vi "Input Items Write.vi"(4 "error in (no error)":errorcluster, 5 "Value":string[](array[string]), 6 "Container State":T4, 7 "Display State In":T1) -> (0 "error out":errorcluster, 3 "Display State Out":T1)   [LabVIEW 2020, in "PXISlotGP.xctl"]
uses:
  PXISlotGP.xctl
  <vilib>/_xctls/Container State.ctl
  State.ctl
  PXISlot XControl/Connector Type.ctl
  AOAIRefs.ctl
  <vilib>/_xctls/XControlSupport.lvlib
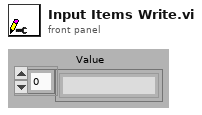
[diagram p1: front panel]
types:
  T1 = typedef "PXISlotGP.xctl/State.ctl" = cluster{"Connector Type":T2, "Hide unused":bool, "Trigger Visible":bool, "TabRef":refnum<vi>, "ConnRefs":refnum<vi>[], "PaneRef":refnum<vi>, "AOAIRefs":T3[], "TriggerRefs":refnum<vi>[], "check data":bool, "Name":string, "Events":cluster{"Type changed":refnum<user-event>}}
  T2 = typedef "Connector Type.ctl" = enum16{"None", "PXI-4461", "BNC-2110", "BNC-2090", "PXIe-4463", "PXIe-4464"}
  T3 = typedef "AOAIRefs.ctl" = cluster{"AORefs":refnum<vi>[], "AIRefs":refnum<vi>[]}
  T4 = typedef "XControlSupport.lvlib/Container State.ctl" = cluster{"Indicator?":bool, "Run Mode?":bool, " Refnum":refnum<vi>}
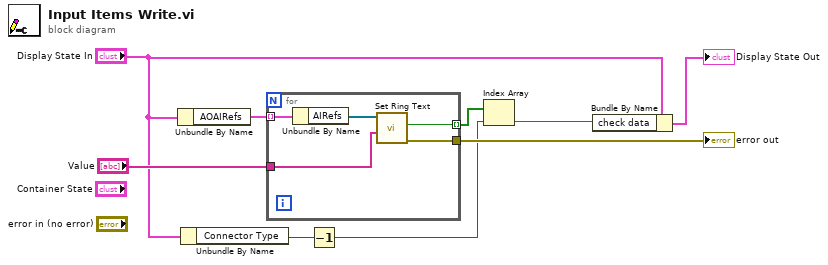
[diagram p0: block diagram]
diagram:
  n1 = Unbundle By Name("Display State In") -> ("AOAIRefs"=w9:T3[])
  n2 = Unbundle By Name("Display State In") -> ("Connector Type"=w3:T2)
  n3 = for {
    tunnel: w9 -> [w14] mode=indexing
    tunnel: "Value" -> [w12]
    tunnel: [w11] -> w7
    tunnel: [w10] -> w4 mode=indexing
    n4 = Unbundle By Name(w14) -> ("AIRefs"=w13:refnum<vi>[])
    n5 = call "Set Ring Text.vi"("Items"=w12, "Rings"=w13) -> ("error out"=w11:errorcluster, "data changed"=w10:bool)  [unwired: 8 in]
  }
  "error out" <- w7
  n6 = Decrement(x=w3) -> (x-1=w1:T2)
  n7 = Index Array(array=w4, index=w1) -> (element=w6:bool)
  n8 = Bundle By Name(cluster="Display State In", "check data"=w6) -> (→"Display State Out":T1)
